vi "ex_FileReadTDMS.vi"(0 "file path in":path, 1 "Read specified segment size":bool, 2 "First time?":bool, 3 "Ask user for file":bool, 4 "Segment Size":i32, 5 "error in (no error)":errorcluster, 6 "Plugin info":T1, 7 "read info in":T2, 9 "single values":bool, 10 "Lock file":bool) -> (13 "read info out":T2, 14 "file path out":path, 15 "Comment":string, 16 "Signals":waveform(dbl)[](array[waveform]), 17 "Description":string, 18 "EOF":bool, 19 "error out":errorcluster)   [LabVIEW 2020]
uses:
  <vilib>/Platform/express/TDMExpress.llb/ex_readInfoTDM.ctl
  <vilib>/Platform/express/TDMExpress.llb/ex_readChannelInfo.ctl
  <vilib>/express/express shared/ExFile.llb/ex_TdmData.ctl
  <vilib>/express/express shared/ExFile.llb/ex_TdmProperty.ctl
  <vilib>/express/express shared/ex_EditUserDefinedProperties/usiDataType.ctl
  <vilib>/express/express shared/ExFile.llb/ex_PluginInfo.ctl
  <vilib>/express/express shared/ExFile.llb/ex_FileGlobals.vi
panel:
  out "*(type *) &x":i32
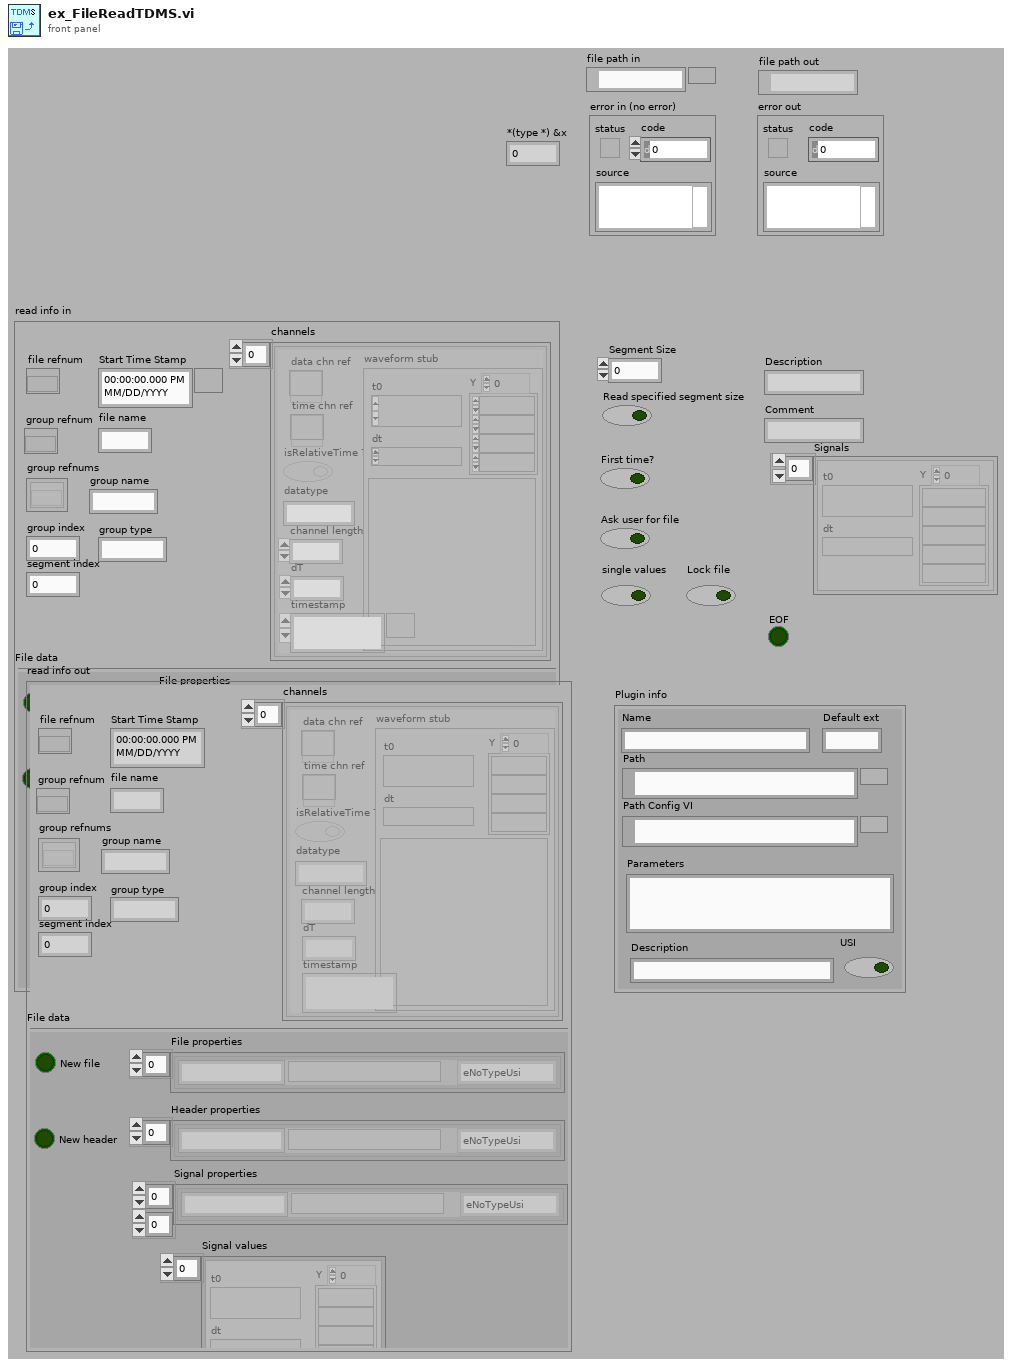
[diagram p1: front panel]
types:
  T1 = typedef "ex_PluginInfo.ctl" = cluster{"Name":string, "Path":path, "Default ext":string, "Parameters":string, "Path Config VI":path, "Description":string, "USI":bool}
  T2 = typedef "ex_readInfoTDM.ctl" = cluster{"file refnum":refnum<k20>, "group refnum":refnum<k20>, "group name":string, "group type":string, "Start Time Stamp":timestamp, "group index":u32, "group refnums":refnum<k20>[], "file name":string, "segment index":u32, "channels":T3[], "File data":T4}
  T3 = typedef "ex_readChannelInfo.ctl" = cluster{"data chn ref":refnum<k20>, "time chn ref":refnum<k20>, "isRelativeTime ?":bool, "channel length":u32, "dT":dbl, "waveform stub":waveform(dbl), "datatype":string, "timestamp":timestamp}
  T4 = typedef "ex_TdmData.ctl" = cluster{"New file":bool, "New header":bool, "File properties":T5[], "Header properties":T5[], "Signal properties":T5[][], "Signal values":waveform(dbl)[]}
  T5 = typedef "ex_TdmProperty.ctl" = cluster{"Name":string, "Type":T6, "Value":variant}
  T6 = typedef "usiDataType.ctl" = enum16{"eNoTypeUsi", "eInt8Usi", "eInt16Usi", "eInt32Usi", "eInt64Usi", "eUInt8Usi", "eUInt16Usi", "eUInt32Usi", "eUInt64Usi", "eFloat32Usi", "eFloat64Usi", "- 0", "- 1", "- 2", "- 3", "- 4", "- 5", "- 6", "- 7", "- 8", "- 9", "eString8Usi", "eString16Usi", "eStringUsi", "eEnumUsi", "- 10", "- 11", "- 12", "- 13", "- 14", "eTimeUsi", "- 15", "- 16", "- 17", "- 18", "- 19", "- 20", "- 21", "- 22", "- 23", "eInstanceUsi", "eStoreUsi"}
  T7 = enum16{"open", "open or create", "create or replace", "create", "open (read-only)"}
  T8 = enum32{"existing file", "new file", "new or existing file", "existing dir", "new dir", "new or existing dir", "existing file (use LLBs)", "new file (use LLBs)", "new or existing file (use LLBs)", "new or existing file or directory (use LLBs)"}
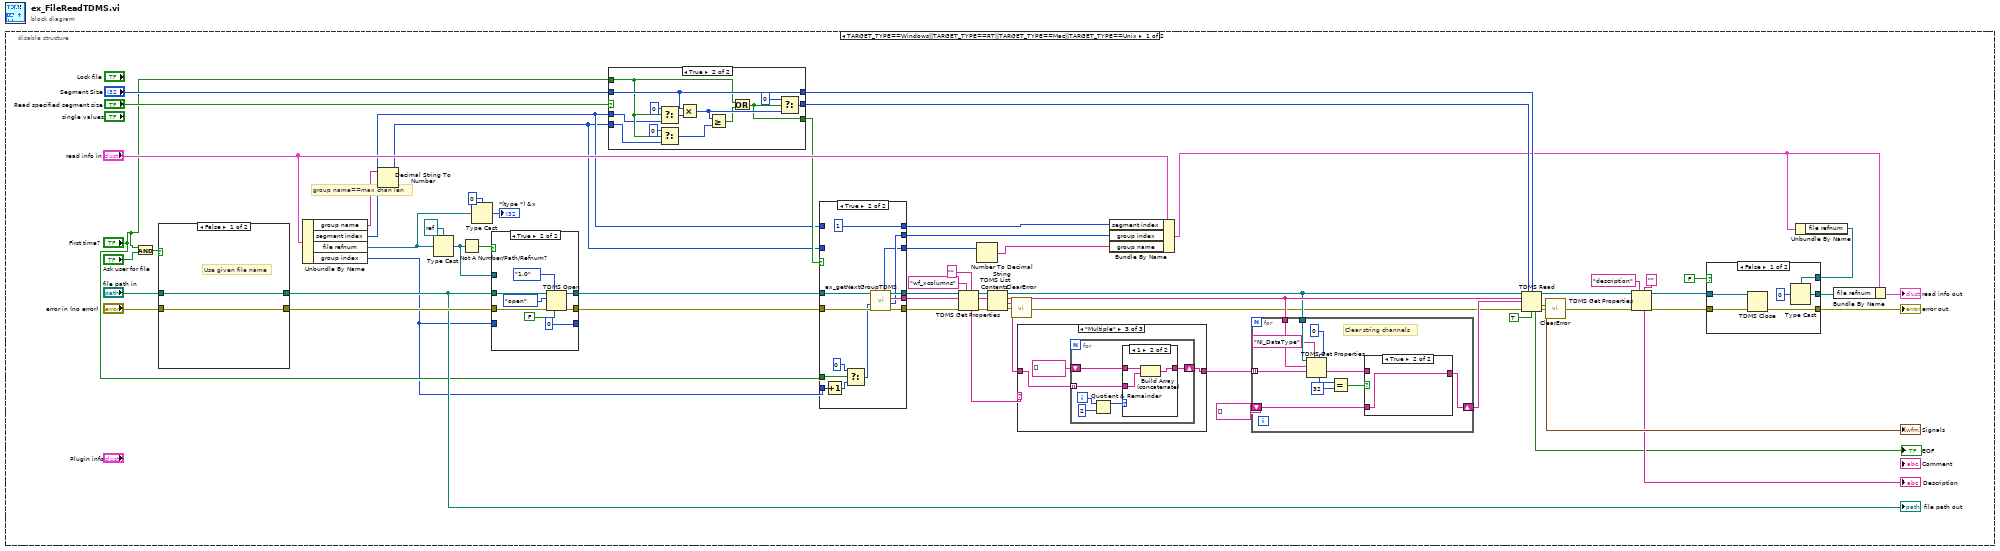
[diagram p0: block diagram]
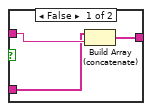
[diagram p2: hidden frame]
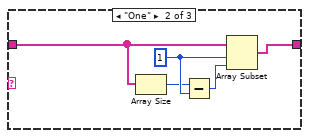
[diagram p4: hidden frame]
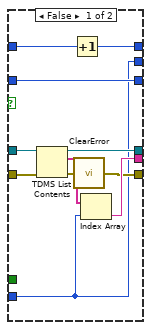
[diagram p6: hidden frame]
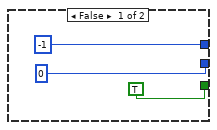
[diagram p7: hidden frame]
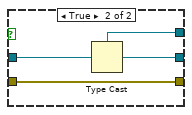
[diagram p9: hidden frame]
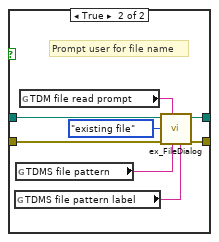
[diagram p10: hidden frame]
diagram:
  n1 = disable-structure shown="TARGET_TYPE==Windows||TARGET_TYPE==RT||TARGET_TYPE==Mac||TARGET_TYPE==Unix" {
    frame condition #0 (active) {
      # "group name==max chan len"
      n2 = And(x="First time?", y="Ask user for file") -> (x .and. y?=w63:bool)
      n3 = case shown="False" w63 {
        tunnel: "file path in" -> [w160 w162]
        tunnel: [w159 w164] -> w59
        tunnel: [w160 w161] -> w49
        tunnel: "error in (no error)" -> [w159 w163]
        frame False {
          # "Use given file name"
        }
        frame True {
          # "Prompt user for file name"
          n4 = global read "ex_FileGlobals.vi" "TDMS file pattern label"() -> (w165:string)
          n5 = global read "ex_FileGlobals.vi" "TDMS file pattern"() -> (w166:string)
          n6 = global read "ex_FileGlobals.vi" "TDM file read prompt"() -> (w167:string)
          n7 = call <vilib>:"ex_FileDialog.vi"("pattern label"=w165, "pattern"=w166, "prompt"=w167, "error in (no error)"=w163, "select mode"=T8."existing file", "start path"=w162) -> ("error out"=w164:errorcluster, "selected file path"=w161:path)  [unwired: 4 out]
        }
      }
      "file path out" <- w49
      n8 = Unbundle By Name("read info in") -> ("group name"=w41:string, "segment index"=w34:u32, "file refnum"=w48:refnum<k20>, "group index"=w30:u32)
      n9 = Decimal String To Number(string=w41) -> (number=w33:i32)  [unwired: 3 out]
      n10 = Type Cast(type=refnum<k34> refnum ("tdms file out"), x=w48) -> (*(type *) &x=w51:refnum<k34>)
      n11 = Not A Number/Path/Refnum?(number/path/refnum=w51) -> (NaN/Path/Refnum?=w54:bool)
      n12 = Type Cast(type=0, x=w48) -> (*(type *) &x=→"*(type *) &x":i32)
      n13 = case shown="True" w54 {
        tunnel: w49 -> [_ w148]
        tunnel: w59 -> [w140 w147]
        tunnel: [w138 w145] -> w36
        tunnel: [w140 w144] -> w35
        tunnel: w51 -> [w138 _]
        tunnel: [w139 0] -> _
        tunnel: w30 -> [w139 _]
        frame False {
        }
        frame True {
          n14 = TDMS Open(6:FALSE ("disable buffering (T)"), 7:enum16{"1.0", "2.0"}."1.0" ("file format version (2.0)"), 8:w147, 10:T7."open" ("operation"), 11:w148) -> (0:w144:errorcluster, 3:w145:refnum<k34>)  [unwired: 2 in]
        }
      }
      n15 = case shown="True" "Read specified segment size" {
        tunnel: "Segment Size" -> [_ w137]
        tunnel: w34 -> [_ w126]
        tunnel: [-1 ("f") w137] -> w39
        tunnel: [u32 0 ("Numeric 2") w134] -> w38
        tunnel: w33 -> [_ w128]
        tunnel: [TRUE w132] -> w37
        tunnel: "First time?" -> [_ w129]
        frame False {
        }
        frame True {
          n16 = Select(t=0, s=w129, f=w126) -> (s? t:f=w125:u32)
          n17 = Select(t=0, s=w129, f=w128) -> (s? t:f=w127:i32)
          n18 = Multiply(x=w137, y=w125) -> (x*y=w135:u32)
          n19 = Greater Or Equal?(x=w135, y=w127) -> (x >= y?=w133:bool)
          n20 = Or(x=w129, y=w133) -> (x .or. y?=w132:bool)
          n21 = Select(t=0, s=w132, f=w135) -> (s? t:f=w134:u32)
        }
      }
      n22 = case shown="True" w37 {
        tunnel: [w101 w121] -> w29
        tunnel: [w102 w120] -> w27
        tunnel: [w108 w119] -> w28
        tunnel: [w100 w118] -> w45
        tunnel: [w107 w117] -> w42
        tunnel: w35 -> [w103 w115]
        tunnel: w36 -> [w104 w114]
        tunnel: w33 -> [w107 _]
        tunnel: w34 -> [w106 _]
        tunnel: [w105 u32 1] -> w32
        tunnel: "First time?" -> [_ w111]
        tunnel: w30 -> [w100 w110]
        frame False {
          n23 = TDMS List Contents(4:w103, 7:w104) -> (0:w98:errorcluster, 2:w99:string[], 3:w101:refnum<k34>)  [unwired: 2 out]
          n24 = Increment(x=w106) -> (x+1=w105:u32)
          n25 = call <vilib>:"ClearError.vi"("error in (no error)"=w98) -> ("error out"=w102:errorcluster)
          n26 = Index Array(array=w99, index=w100) -> (element=w108:string)
        }
        frame True {
          n27 = Increment(x=w110) -> (x+1=w112:u32)
          n28 = Select(t=0, s=w111, f=w112) -> (s? t:f=w109:u32)
          n29 = call <vilib>:"ex_getNextGroupTDMS.vi"("error in (no error)"=w115, "group index in"=w109, "tdms file in"=w114) -> ("error out"=w120:errorcluster, "group index out"=w118:u32, "group name"=w119:string, "tdms file out"=w121:refnum<k34>, "max len"=w117:i32)  [unwired: 4 out]
        }
      }
      n30 = TDMS Get Properties(5:"" ("data type"), 7:"wf_xcolumns" ("property name"), 8:w27, 10:w28, 11:w29) -> (0:w26:errorcluster, 2:w25:string, 3:w24:refnum<k34>, 4:w21:string)  [unwired: 3 out]
      n31 = Number To Decimal String(number=w42) -> (decimal integer string=w43:string)  [unwired: 1 out]
      n32 = TDMS List Contents(4:w26, 6:w25, 7:w24) -> (0:w1:errorcluster, 1:w6:string[], 2:w19:string, 3:w14:refnum<k34>)
      n33 = call <vilib>:"ClearError.vi"("error in (no error)"=w1) -> ("error out"=w13:errorcluster)
      n34 = case shown="\"Multiple\"" w21 {
        tunnel: [w79 w84 w85] -> w20
        tunnel: w6 -> [w79 w83 w87]
        frame Default {
        }
        frame "One" {
          w82 = 1 ("index")
          n35 = Array Size(array=w83) -> (size(s)=w81:i32)
          n36 = Subtract(x=w81, y=w82) -> (x-y=w80:i32)
          n37 = Array Subset(array=w83, index=w82, length=w80) -> (w84:string[])
        }
        frame "Multiple" {
          n38 = for {
            shift-right: [w90] -> w85
            shift-left: string[] [] -> [w91]
            tunnel: w87 -> [w89] mode=indexing
            i -> [w93]
            n39 = Quotient & Remainder(x=w93, y=2) -> (x-y*floor(x/y)=w88:i32)  [unwired: 1 out]
            n40 = case shown="1" w88 {
              tunnel: w91 -> [w94 w97]
              tunnel: [w94 w96] -> w90
              tunnel: w89 -> [_ w95]
              frame 0, Default {
              }
              frame 1 {
                n41 = Build Array (concatenate)(w97, w95) -> (w96:string[])
              }
            }
          }
        }
      }
      n42 = Bundle By Name(cluster="read info in", "segment index"=w32, "group index"=w45, "group name"=w43) -> (w3:T2)
      n43 = for {
        tunnel: w20 -> [w72] mode=indexing
        tunnel: w14 -> [w74]
        tunnel: w19 -> [w73]
        shift-right: [w67] -> w17
        shift-left: string[] [] -> [w66]
        # "Clear string channels"
        n44 = TDMS Get Properties(5:0, 7:"NI_DataType" ("property name"), 9:w72, 10:w73, 11:w74) -> (1:w68:string, 4:w70:i32)  [unwired: 1 in, 4 out]
        n45 = Equal?(x=w70, y=32) -> (x = y?=w69:bool)
        n46 = case shown="True" w69 {
          tunnel: w68 -> [w76 _]
          tunnel: w66 -> [w75 w78]
          tunnel: [w77 w78] -> w67
          frame False {
            n47 = Build Array (concatenate)(w75, w76) -> (w77:string[])
          }
          frame True {
          }
        }
      }
      n48 = TDMS Read(0:w14, 1:w38, 2:w39, 5:w19, 7:w17, 11:w13, 13:TRUE ("return channels in file order? (F)")) -> (4:w12:refnum<k34>, 10:→"Signals":waveform(dbl)[], 14:→"EOF":bool, 15:w7:errorcluster)  [unwired: 1 in, 2 out]
      n49 = call <vilib>:"ClearError.vi"("error in (no error)"=w7) -> ("error out"=w11:errorcluster)
      n50 = TDMS Get Properties(5:"" ("data type"), 7:"description" ("property name"), 8:w11, 11:w12) -> (0:w9:errorcluster, 3:w10:refnum<k34>, 4:→"Description":string)  [unwired: 5 out]
      n51 = Unbundle By Name(w3) -> ("file refnum"=w2:refnum<k20>)
      n52 = case shown="False" FALSE {
        tunnel: w10 -> [w154 w157]
        tunnel: w9 -> [w152 w158]
        tunnel: [w153 w158] -> w58
        tunnel: [w151 w156] -> w56
        tunnel: w2 -> [w150 w155]
        frame False {
          n53 = TDMS Close(8:w152, 11:w154) -> (0:w153:errorcluster)  [unwired: 1 out]
          n54 = Type Cast(type=w150, x=0) -> (*(type *) &x=w151:refnum<k20>)
        }
        frame True {
          n55 = Type Cast(type=w155, x=w157) -> (*(type *) &x=w156:refnum<k20>)
        }
      }
      "error out" <- w58
      n56 = Bundle By Name(cluster=w3, "file refnum"=w56) -> (→"read info out":T2)
    }
    frame condition #1 {
    }
  }
